vi "FitSineWave.vi"(8 "error in (no error)":errorcluster, 9 "Bin Size (3)":i32=3, 10 "N Sigma (6)":dbl=6.0 format="%#_13g", 11 "Power Graph":cluster{dbl[], dbl[]}(graph)) -> (0 "error out":errorcluster, 2 "best fit parameters":dbl[](array[numeric]), 3 "Power Graph 2":cluster{dbl[], "best nonlinear fit":dbl[]}[](graph))   [LabVIEW 2019]
uses:
  <vilib>/gmath/NumericalOptimization/Nonlinear Curve Fit LM formula string.vi
  <vilib>/gmath/NI_Gmath.lvlib
panel:
  in  "initial parameters":dbl[](array[numeric])=[100.0, 1.2, 0.06]
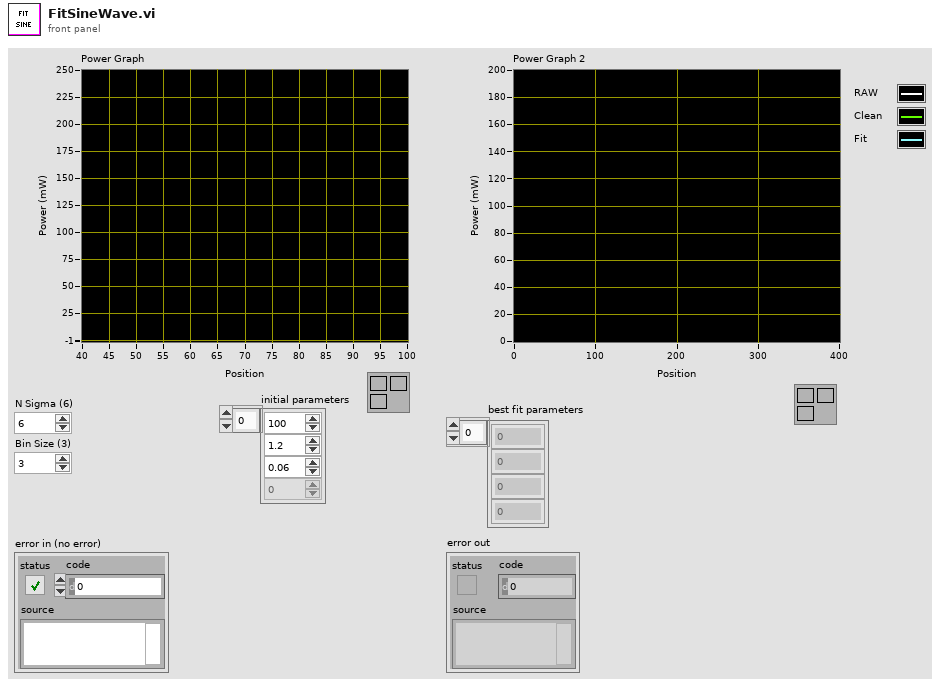
[diagram p1: front panel]
types:
  T1 = cluster{"model":string, "Parameters":string[], "x":string}
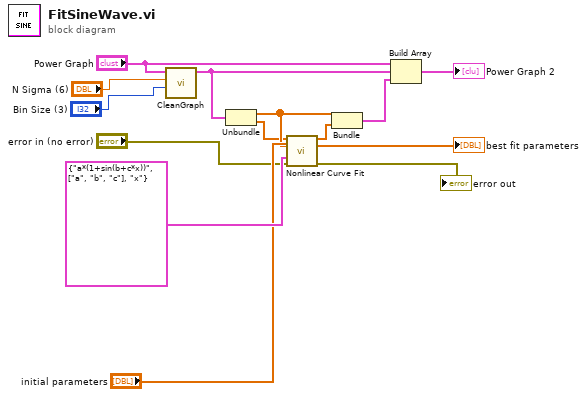
[diagram p0: block diagram]
diagram:
  n1 = call "CleanGraph.vi"("Bin Size"="Bin Size (3)", "N Sigma"="N Sigma (6)", "XY Graph In"="Power Graph") -> ("XY Graph Out"=w4:cluster{dbl[], dbl[]})  [unwired: 8 in]
  n2 = Unbundle(w4) -> (w7:dbl[], w6:dbl[])
  n3 = call-poly <vilib>:"Nonlinear Curve Fit.vi"("Y"=w6, "initial parameters"="initial parameters", "X"=w7, "model description"=T1 {"model"="a*(1+sin(b+c*x))", "Parameters"=["a", "b", "c"], "x"="x"}, "error in (no error)"="error in (no error)") -> ("best nonlinear fit"=w11:dbl[], "best fit parameters"=→"best fit parameters":dbl[], "error out"=→"error out":errorcluster)  [unwired: 6 in, 2 out]
  n4 = Bundle(w7, "best nonlinear fit"=w11) -> (w10:cluster{dbl[], "best nonlinear fit":dbl[]})  [unwired: 1 in]
  n5 = Build Array("Power Graph", w4, w10) -> (→"Power Graph 2":cluster{dbl[], "best nonlinear fit":dbl[]}[])
